vi "Get Backpressure Name.vi"(3 "Parent Name":string) -> (5 "Backpressure Name":string)   [LabVIEW 2021, in "CIF_NI_CIPC.lvlib"]
uses:
  CIF_NI_CIPC.lvlib
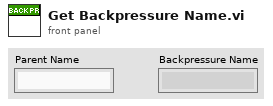
[diagram p1: front panel]
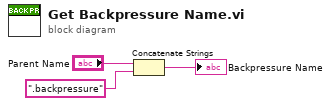
[diagram p0: block diagram]
diagram:
  n1 = Concatenate Strings("Parent Name", ".backpressure" ("string")) -> (→"Backpressure Name":string)
